vi "A-B Fit.vi"(1 "B":dbl[][](graph)=array90x900[81000 elements], 2 "A":dbl[][](graph)=array90x900[81000 elements]) -> (0 "|A-B|":dbl)   [LabVIEW 2016]
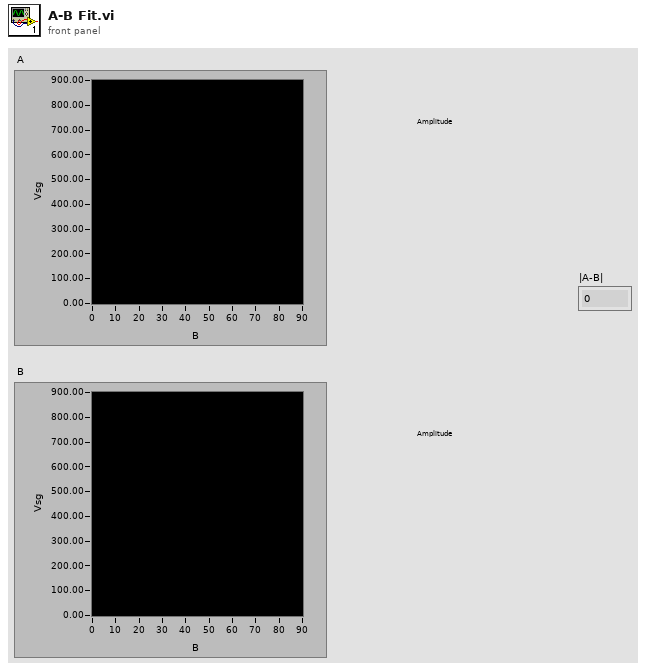
[diagram p1: front panel]
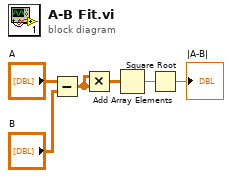
[diagram p0: block diagram]
diagram:
  n1 = Subtract(x="A", y="B") -> (x-y=w4:dbl[][])
  n2 = Multiply(x=w4, y=w4) -> (x*y=w3:dbl[][])
  n3 = Add Array Elements(numeric array=w3) -> (sum=w2:dbl)
  n4 = Square Root(x=w2) -> (sqrt(x)=→"|A-B|":dbl)
